vi "Wait n mSec.vi"(0 "error in (no error)":errorcluster, 1 "milliseconds to wait (500)":u32=500) -> (2 "error out":errorcluster)   [LabVIEW 2019]
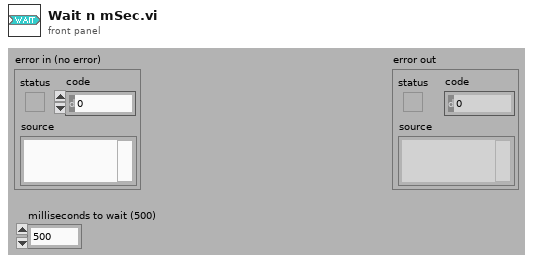
[diagram p1: front panel]
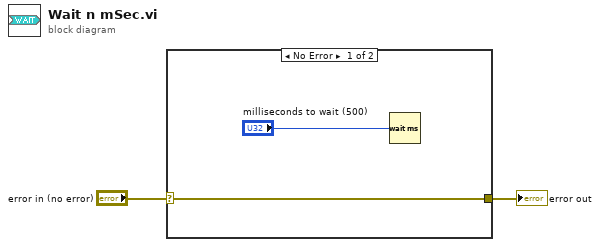
[diagram p0: block diagram]
diagram:
  n1 = case shown="No Error" "error in (no error)" {
    selector: "error in (no error)" -> [w4 w5]
    tunnel: [w4 w5] -> w1
    frame No Error {
      n2 = Wait (ms)(milliseconds to wait="milliseconds to wait (500)") -> ()  [unwired: 1 out]
    }
    frame Error {
    }
  }
  "error out" <- w1
